vi "get_plugins.vi"() -> ()   [LabVIEW 2010]
panel:
  in  "stop":bool
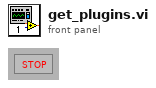
[diagram p1: front panel]
types:
  T1 = enum32{"Invalid", "Standard", "Closed", "Hidden", "Minimized", "Maximized"}
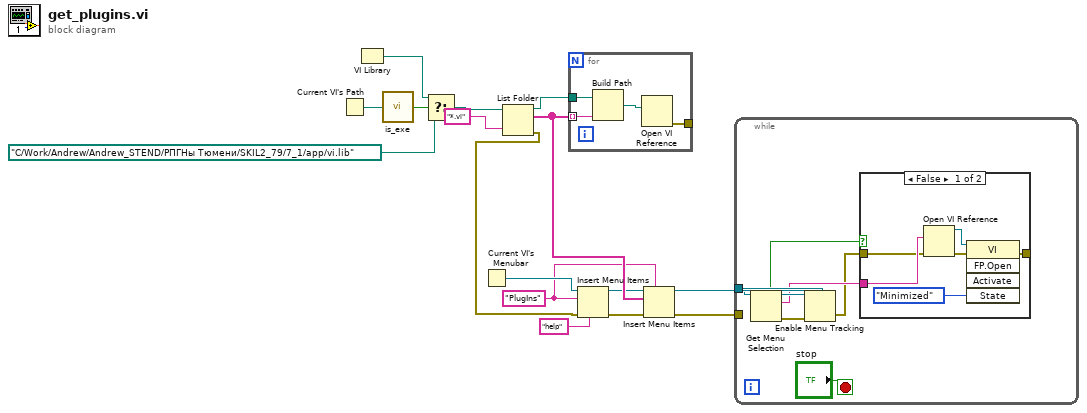
[diagram p0: block diagram]
diagram:
  w7 = "PlugIns" ("menu tag")
  n1 = Current VI's Path() -> (path=w16:path)
  n2 = VI Library() -> (path=w14:path)
  n3 = call "is_exe.vi"("path"=w16) -> ("exe?"=w15:bool)  [unwired: 2 in, 2 out]
  n4 = Select(t=w14, s=w15, f=path "C:/Work/Andrew/Andrew_STEND/РПГНы Тюмени/SKIL2_79/7_1/app/vi.lib") -> (s? t:f=w13:path)
  n5 = Current VI's Menubar() -> (w10:refnum<k9>)
  n6 = List Folder(path=w13, pattern="*.vi") -> (path out=w4:path, filenames=w8:string[], error out=w2:errorcluster)  [unwired: 2 in, 1 out]
  n7 = for {
    tunnel: w8 -> [w20] mode=indexing
    tunnel: w4 -> [w19]
    tunnel: [w17] -> _
    n8 = Build Path(base path=w19, name or relative path=w20) -> (appended path=w18:path)
    n9 = Open VI Reference(vi path=w18) -> (error out=w17:errorcluster)  [unwired: 5 in, 1 out]
  }
  n10 = Insert Menu Items(4:"help" ("after item"), 6:w2, 8:w7, 9:w10) -> (0:w6:errorcluster, 3:w5:refnum<k9>)  [unwired: 2 in, 1 out]
  n11 = Insert Menu Items(5:w7, 6:w6, 8:w8, 9:w5) -> (0:w1:errorcluster, 3:w3:refnum<k9>)  [unwired: 2 in, 1 out]
  n12 = while {
    tunnel: w3 -> [w26]
    tunnel: w1 -> [_]
    stop <- "stop" stop-if-true
    n13 = Get Menu Selection(0:w26) -> (4:w22:bool, 5:w24:refnum<k9>, 6:w23:string, 8:w25:errorcluster)  [unwired: 3 in, 1 out]
    n14 = Enable Menu Tracking(2:w25, 4:w24) -> (0:w21:errorcluster)  [unwired: 1 in, 1 out]
    n15 = case shown="False" w22 {
      tunnel: w23 -> [w31 _]
      tunnel: w21 -> [w29 w34]
      tunnel: [w28 w34] -> _
      frame False {
        n16 = Open VI Reference(vi path=w31, error in (no error)=w29) -> (vi reference=w32:refnum<vi>, error out=w30:errorcluster)  [unwired: 4 in]
        n17 = invoke class="VI" method="FP.Open"(reference=w32, error in=w30, "State"=T1."Minimized") -> (error out=w28:errorcluster)  [unwired: 2 in, 4 out]
      }
      frame True {
      }
    }
  }
